vi "RobotDriveMotors.vi"(8 "error in (no error)":errorcluster, 9 "RightSpeed":dbl, 10 "LeftSpeed":dbl, 11 "RobotDriveDevRef":T1={"DevStatus"={"status"=FALSE, "code"=0, "source"=""}, "Motors[]"=[], "Square Inputs"=FALSE, "Max Output"=1.0}) -> (0 "error out":errorcluster, 2 "Motor Values":dbl[](array[numeric]), 3 "RobotDriveDevRef":T1={"DevStatus"={"status"=FALSE, "code"=0, "source"=""}, "Motors[]"=[], "Square Inputs"=FALSE, "Max Output"=1.0})   [LabVIEW 2016]
doc: "Determines the motor configuration and sends the speed values to the appropriate motors.\n\nThis software is licensed. Open the labview\\readme\\WPI Robotics Library Open Source License.txt file for more information."
uses:
  <vilib>/Rock Robotics/WPI/RobotDrive/WPI_RobotDriveDevRef.ctl
  <vilib>/Rock Robotics/WPI/MotorControl/WPI_MotorControlDeviceRef.ctl
  <vilib>/Rock Robotics/WPI/MotorControl/WPI_MotorControlType.ctl
  <vilib>/Rock Robotics/SystemInterfaces/DIO/FPGA_DIOPWMChannel.ctl
  <vilib>/Rock Robotics/WPI/PWM/WPI_PWMDeadband.ctl
  <vilib>/Rock Robotics/WPI/RobotDrive/WPI_RobotDriveMotorSelectorEnum.ctl
  RobotDriveMotorSelectorEnum.ctl
  <vilib>/Rock Robotics/WPI/RobotDrive/WPI_RobotDriveSafetyCheck.vi
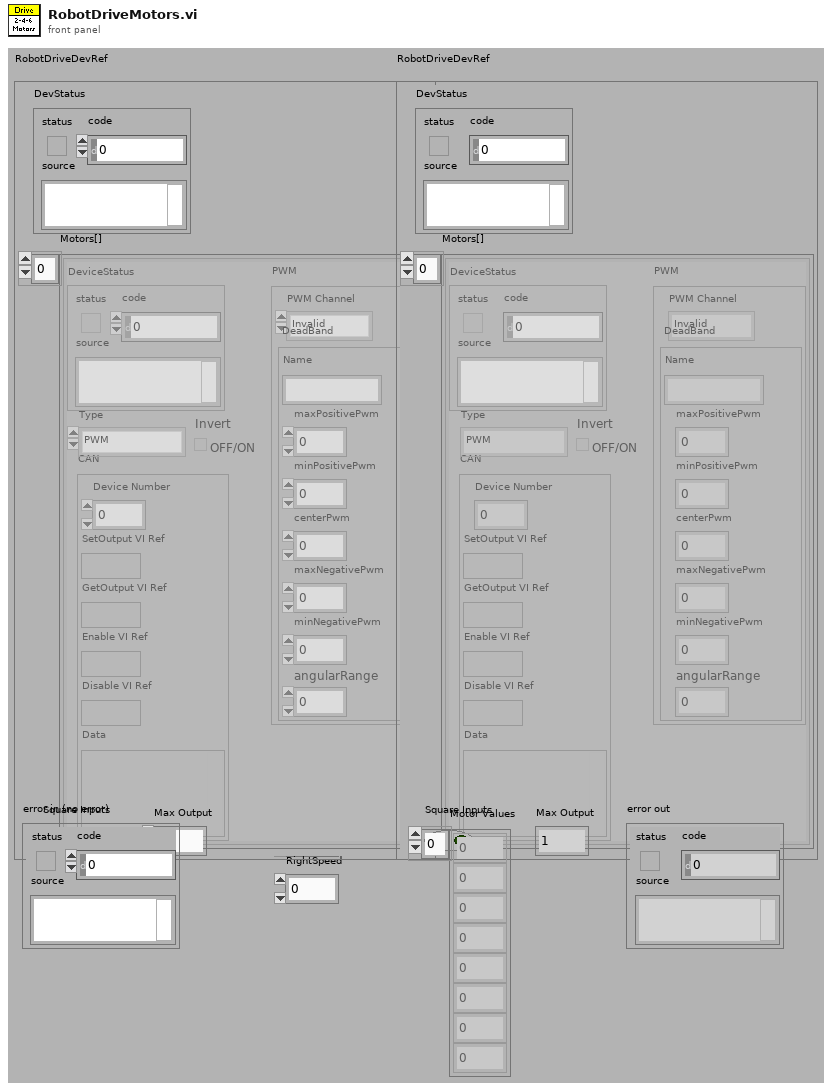
[diagram p1: front panel]
types:
  T1 = typedef "WPI_RobotDriveDevRef.ctl" = cluster{"DevStatus":errorcluster, "Motors[]":T2[], "Square Inputs":bool, "Max Output":dbl}
  T2 = typedef "WPI_MotorControlDeviceRef.ctl" = cluster{"DeviceStatus":errorcluster, "Type":T3, "PWM":cluster{"PWM Channel":T4, "DeadBand":T5}, "CAN":cluster{"Device Number":u8, "SetOutput VI Ref":variant, "GetOutput VI Ref":variant, "Enable VI Ref":variant, "Disable VI Ref":variant, "Data":variant}, "Invert":bool}
  T3 = typedef "WPI_MotorControlType.ctl" = enum16{"PWM", "CAN"}
  T4 = typedef "FPGA_DIOPWMChannel.ctl" = enum8{"PWM 0", "PWM 1", "PWM 2", "PWM 3", "PWM 4", "PWM 5", "PWM 6", "PWM 7", "PWM 8", "PWM 9", "PWM MXP 0", "PWM MXP 1", "PWM MXP 2", "PWM MXP 3", "PWM MXP 4", "PWM MXP 5", "PWM MXP 6", "PWM MXP 7", "PWM MXP 8", "PWM MXP 9", "Invalid"}
  T5 = typedef "WPI_PWMDeadband.ctl" = cluster{"Name":string, "maxPositivePwm":i32, "minPositivePwm":i32, "centerPwm":i32, "maxNegativePwm":i32, "minNegativePwm":i32, "angularRange":u16}
  T6 = typedef "WPI_RobotDriveMotorSelectorEnum.ctl" = enum16{"Rear Left Motor", "Rear Right Motor", "Front Left Motor", "Front Right Motor"}
  T7 = typedef "RobotDriveMotorSelectorEnum.ctl" = enum16{"Left Motor 1", "Right Motor 1", "Left Motor 2", "Right Motor 2", "Left Motor 3", "Right Motor 3"}
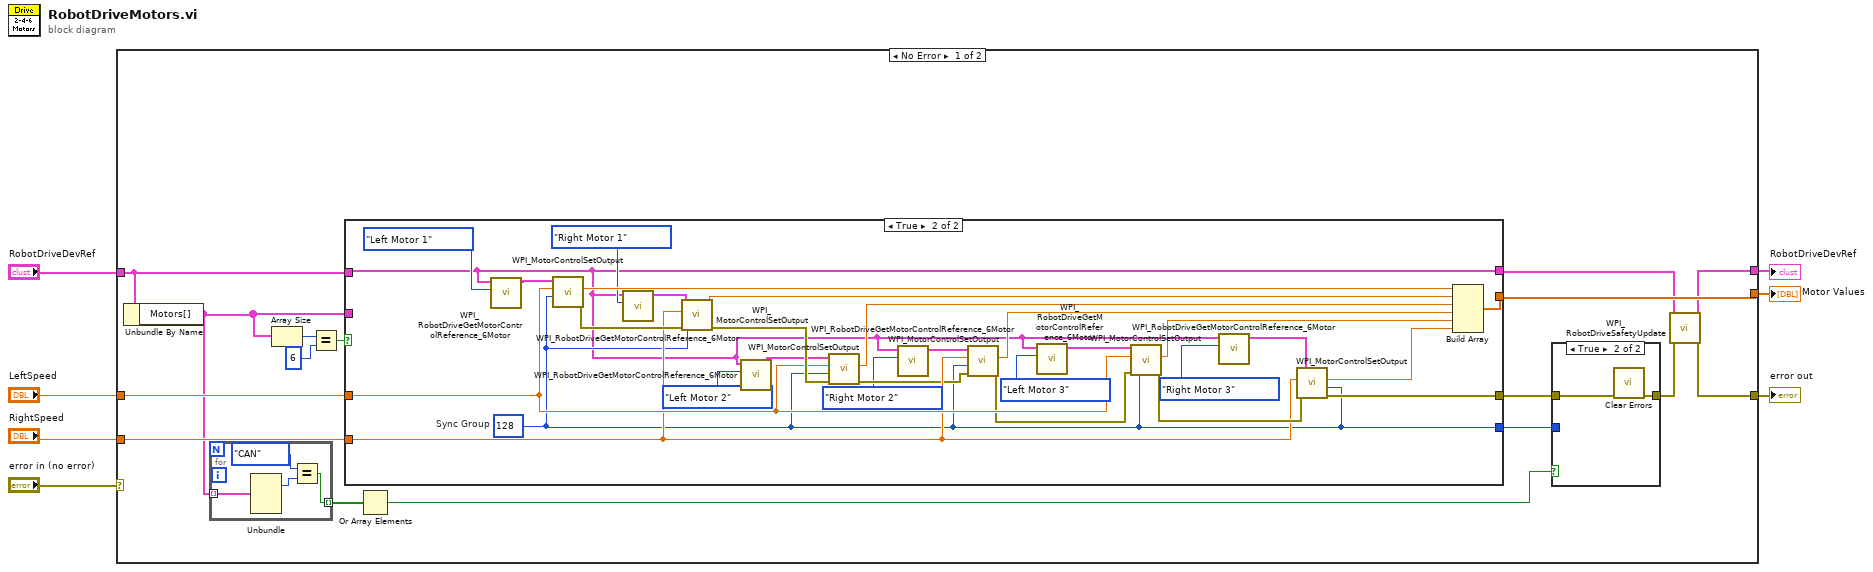
[diagram p0: block diagram]
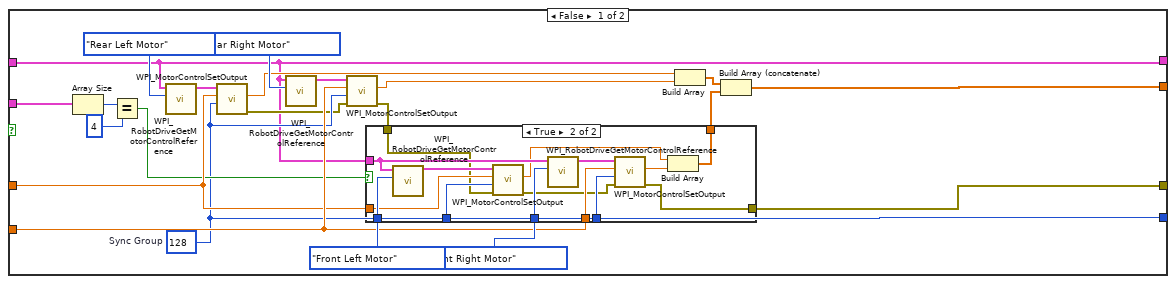
[diagram p2: hidden frame]
diagram:
  n1 = case shown="No Error" "error in (no error)" {
    selector: "error in (no error)" -> [_ w99]
    tunnel: "RobotDriveDevRef" -> [w23 w98]
    tunnel: [w13 w98] -> w6
    tunnel: "LeftSpeed" -> [w21 _]
    tunnel: "RightSpeed" -> [w22 _]
    tunnel: [w14 w99] -> w2
    tunnel: [w16 _] -> w1
    frame No Error {
      n2 = Unbundle By Name(w23) -> ("Motors[]"=w9:T2[])
      n3 = for {
        tunnel: w9 -> [w94] mode=indexing
        tunnel: [w91] -> w19 mode=indexing
        n4 = Unbundle(w94) -> ("Type"=w93:T3)  [unwired: 4 out]
        n5 = Equal?(x=enum16{"PWM", "CAN"}."CAN" ("Type"), y=w93) -> (x = y?=w91:bool)
      }
      n6 = Array Size(array=w9) -> (size(s)=w11:i32)
      n7 = Equal?(x=w11, y=6) -> (x = y?=w8:bool)
      n8 = case shown="True" w8 {
        tunnel: w23 -> [w24 w63]
        tunnel: w22 -> [w37 w85]
        tunnel: w21 -> [w36 w86]
        tunnel: [w34 w75] -> w20
        tunnel: w9 -> [w33 _]
        tunnel: [w31 w82] -> w17
        tunnel: [w25 w88] -> w16
        tunnel: [w24 w63] -> w12
        frame False {
          w34 = u8 128  # Sync Group
          n9 = Array Size(array=w33) -> (size(s)=w45:i32)
          n10 = Equal?(x=w45, y=4) -> (x = y?=w35:bool)
          n11 = call <vilib>:"WPI_RobotDriveGetMotorControlReference.vi"("MotorIndex"=WPI_RobotDriveMotorSelectorEnum."Rear Left Motor", "RobotDriveDevRef"=w24) -> ("MotorControlDeviceRef"=w42:T2)  [unwired: 9 out]
          n12 = call <vilib>:"WPI_MotorControlSetOutput.vi"("options"=w34, "Output"=w36, "MotorControlDevRef"=w42) -> ("error out"=w32:errorcluster, "Motor Output"=w29:dbl)  [unwired: 2 in, 5 out]
          n13 = call <vilib>:"WPI_RobotDriveGetMotorControlReference.vi"("MotorIndex"=WPI_RobotDriveMotorSelectorEnum."Rear Right Motor", "RobotDriveDevRef"=w24) -> ("MotorControlDeviceRef"=w43:T2)  [unwired: 9 out]
          n14 = call <vilib>:"WPI_MotorControlSetOutput.vi"("error in (no error)"=w32, "options"=w34, "Output"=w37, "MotorControlDevRef"=w43) -> ("error out"=w30:errorcluster, "Motor Output"=w28:dbl)  [unwired: 1 in, 5 out]
          n15 = case shown="True" w35 {
            tunnel: WPI_RobotDriveMotorSelectorEnum."Front Left Motor" ("MotorIndex") -> [_ w61]
            tunnel: WPI_RobotDriveMotorSelectorEnum."Front Right Motor" ("MotorIndex") -> [_ w60]
            tunnel: w24 -> [_ w59]
            tunnel: w34 -> [_ w58]
            tunnel: w37 -> [_ w57]
            tunnel: w36 -> [_ w56]
            tunnel: [w46 w52] -> w31
            tunnel: w34 -> [_ w53]
            tunnel: w30 -> [w46 w50]
            tunnel: [_ w47] -> w27
            frame False {
            }
            frame True {
              n16 = call <vilib>:"WPI_RobotDriveGetMotorControlReference.vi"("MotorIndex"=w61, "RobotDriveDevRef"=w59) -> ("MotorControlDeviceRef"=w54:T2)  [unwired: 9 out]
              n17 = call <vilib>:"WPI_MotorControlSetOutput.vi"("error in (no error)"=w50, "options"=w53, "Output"=w56, "MotorControlDevRef"=w54) -> ("error out"=w51:errorcluster, "Motor Output"=w48:dbl)  [unwired: 1 in, 5 out]
              n18 = call <vilib>:"WPI_RobotDriveGetMotorControlReference.vi"("MotorIndex"=w60, "RobotDriveDevRef"=w59) -> ("MotorControlDeviceRef"=w55:T2)  [unwired: 9 out]
              n19 = call <vilib>:"WPI_MotorControlSetOutput.vi"("error in (no error)"=w51, "options"=w58, "Output"=w57, "MotorControlDevRef"=w55) -> ("error out"=w52:errorcluster, "Motor Output"=w49:dbl)  [unwired: 1 in, 5 out]
              n20 = Build Array(w48, w49) -> (w47:dbl[])
            }
          }
          n21 = Build Array(w29, w28) -> (w26:dbl[])
          n22 = Build Array (concatenate)(w26, w27) -> (w25:dbl[])
        }
        frame True {
          w75 = u8 128  # Sync Group
          n23 = call "WPI_RobotDriveGetMotorControlReference_6Motor.vi"("Motor Selector Enum"=RobotDriveMotorSelectorEnum."Left Motor 1", "RobotDriveDevRef"=w63) -> ("MotorControlDeviceRef"=w74:T2)  [unwired: 9 in]
          n24 = call <vilib>:"WPI_MotorControlSetOutput.vi"("options"=w75, "Output"=w86, "MotorControlDevRef"=w74) -> ("error out"=w90:errorcluster, "Motor Output"=w81:dbl)  [unwired: 2 in, 5 out]
          n25 = call "WPI_RobotDriveGetMotorControlReference_6Motor.vi"("Motor Selector Enum"=RobotDriveMotorSelectorEnum."Right Motor 1", "RobotDriveDevRef"=w63) -> ("MotorControlDeviceRef"=w72:T2)  [unwired: 9 in]
          n26 = call <vilib>:"WPI_MotorControlSetOutput.vi"("error in (no error)"=w90, "options"=w75, "Output"=w85, "MotorControlDevRef"=w72) -> ("error out"=w89:errorcluster, "Motor Output"=w80:dbl)  [unwired: 1 in, 5 out]
          n27 = call "WPI_RobotDriveGetMotorControlReference_6Motor.vi"("Motor Selector Enum"=RobotDriveMotorSelectorEnum."Left Motor 2", "RobotDriveDevRef"=w63) -> ("MotorControlDeviceRef"=w70:T2)  [unwired: 9 in]
          n28 = call <vilib>:"WPI_MotorControlSetOutput.vi"("error in (no error)"=w89, "options"=w75, "Output"=w86, "MotorControlDevRef"=w70) -> ("error out"=w84:errorcluster, "Motor Output"=w79:dbl)  [unwired: 1 in, 5 out]
          n29 = call "WPI_RobotDriveGetMotorControlReference_6Motor.vi"("Motor Selector Enum"=RobotDriveMotorSelectorEnum."Right Motor 2", "RobotDriveDevRef"=w63) -> ("MotorControlDeviceRef"=w68:T2)  [unwired: 9 in]
          n30 = call <vilib>:"WPI_MotorControlSetOutput.vi"("error in (no error)"=w84, "options"=w75, "Output"=w85, "MotorControlDevRef"=w68) -> ("error out"=w83:errorcluster, "Motor Output"=w78:dbl)  [unwired: 1 in, 5 out]
          n31 = call "WPI_RobotDriveGetMotorControlReference_6Motor.vi"("Motor Selector Enum"=RobotDriveMotorSelectorEnum."Left Motor 3", "RobotDriveDevRef"=w63) -> ("MotorControlDeviceRef"=w66:T2)  [unwired: 9 in]
          n32 = call <vilib>:"WPI_MotorControlSetOutput.vi"("error in (no error)"=w83, "options"=w75, "Output"=w86, "MotorControlDevRef"=w66) -> ("error out"=w87:errorcluster, "Motor Output"=w77:dbl)  [unwired: 1 in, 5 out]
          n33 = call "WPI_RobotDriveGetMotorControlReference_6Motor.vi"("Motor Selector Enum"=RobotDriveMotorSelectorEnum."Right Motor 3", "RobotDriveDevRef"=w63) -> ("MotorControlDeviceRef"=w64:T2)  [unwired: 9 in]
          n34 = call <vilib>:"WPI_MotorControlSetOutput.vi"("error in (no error)"=w87, "options"=w75, "Output"=w85, "MotorControlDevRef"=w64) -> ("error out"=w82:errorcluster, "Motor Output"=w76:dbl)  [unwired: 1 in, 5 out]
          n35 = Build Array(w81, w80, w79, w78, w77, w76) -> (w88:dbl[])
        }
      }
      n36 = Or Array Elements(Boolean array=w19) -> (logical OR=w18:bool)
      n37 = case shown="True" w18 {
        tunnel: w17 -> [w95 w96]
        tunnel: w20 -> [_ _]
        tunnel: [w95 w97] -> w15
        frame False {
        }
        frame True {
          n38 = call <vilib>:"Clear Errors.vi"("error in (no error)"=w96) -> ("error out"=w97:errorcluster)  [unwired: 1 in, 5 out]
        }
      }
      n39 = call <vilib>:"WPI_RobotDriveSafetyUpdate.vi"("error in (no error)"=w15, "RobotDriveDevRef"=w12) -> ("error out"=w14:errorcluster, "RobotDriveDevRef"=w13:T1)  [unwired: 8 out]
    }
    frame Error {
    }
  }
  "RobotDriveDevRef" <- w6
  "error out" <- w2
  "Motor Values" <- w1
